vi "html Header.vi"(4 "Test Result":bool, 6 "Test Operator":string="sna001", 7 "Company":string="ELEMASTER", 8 "Serial Numbe (SN)":string="SN123456789", 9 "Hardware Revision":string="v1.1", 10 "Product Info":string="Power Board", 11 "Product Name":string="Safe Torque Off") -> (3 "html string":string="<!DOCTYPE html>\n<html>\n<head>\n<style>\ntable {\n  font-family: arial, sans-serif;\n  border-collapse: collapse;\n  width: 85%;\n}\n\ntd, th {\n  border: 1px solid #dddddd;\n  text-align: left;\n  padding: 8px;\n}\n\ntr:nth-child(even) {\n  background-color: #dddddd;\n}\n</style>\n</head>\n<body>\r<h1 style=\"background-color:Orange; text-align:center; width:85%\">ELEMASTER-Ro: Test Report</h1> \r<h3 style=\"color:Blue\">Under Test (UUT): Info</h3>   \r<table style=\"width: 50%\">  <tr>\n    <th>Company</th>\n    <th>ADB SAFEGATE</th>\n  </tr>  <tr>\n    <td>Product Name</td>\n    <th>ADB LED LMS</th>\n  </tr>  <tr>\n    <td>Product Info</td>\n    <td>LMS Single</td>\n  </tr>  <tr>\n    <td>Hardware Revision</td>\n    <td>v1.1</td>\n  </tr>  <tr>\n    <td>Serial number (SN)</td>\n    <th>sn:12345</th>\n  </tr>  <tr>\n    <td>Test Operator</td>\n    <td>---</td>\n  </tr>  <tr>\n    <td>Date / Time</td>\n    <td>22/09/2021 / 15:30</td>\n  </tr>   <tr>\n    <th>Test Result</th>\n    <th style=\"background-color:Red;color:White\">FALSE</th>\n  </tr></table>\n</body>\n</html>")   [LabVIEW 2018]
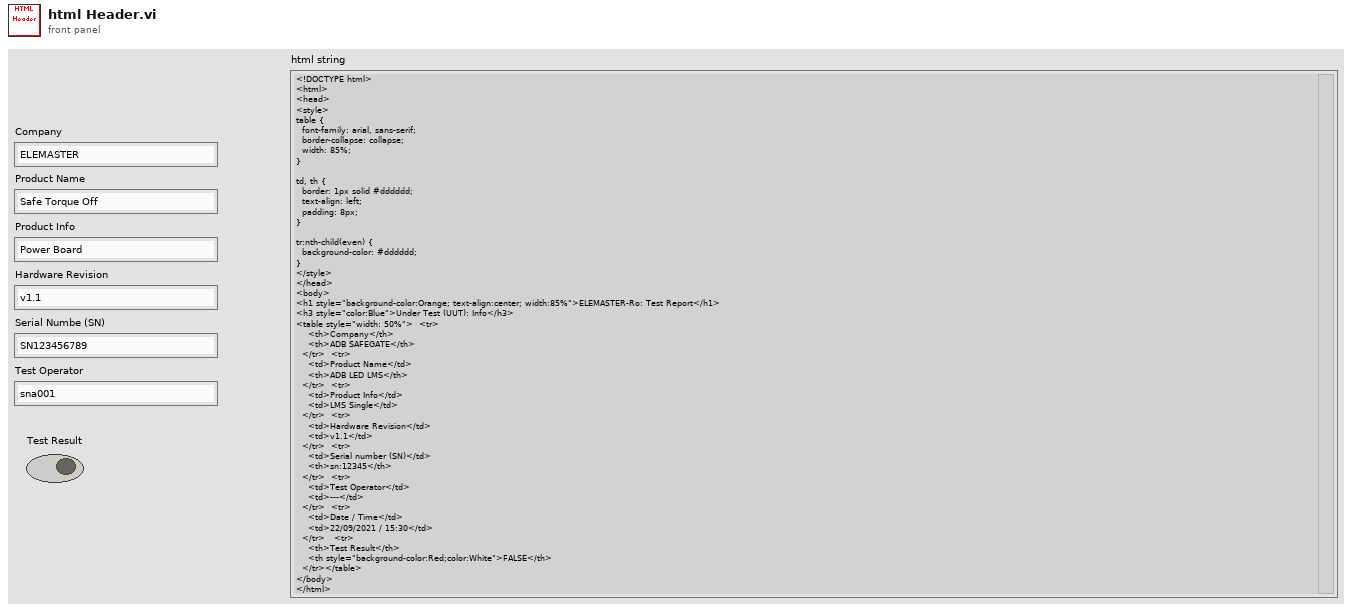
[diagram p1: front panel]
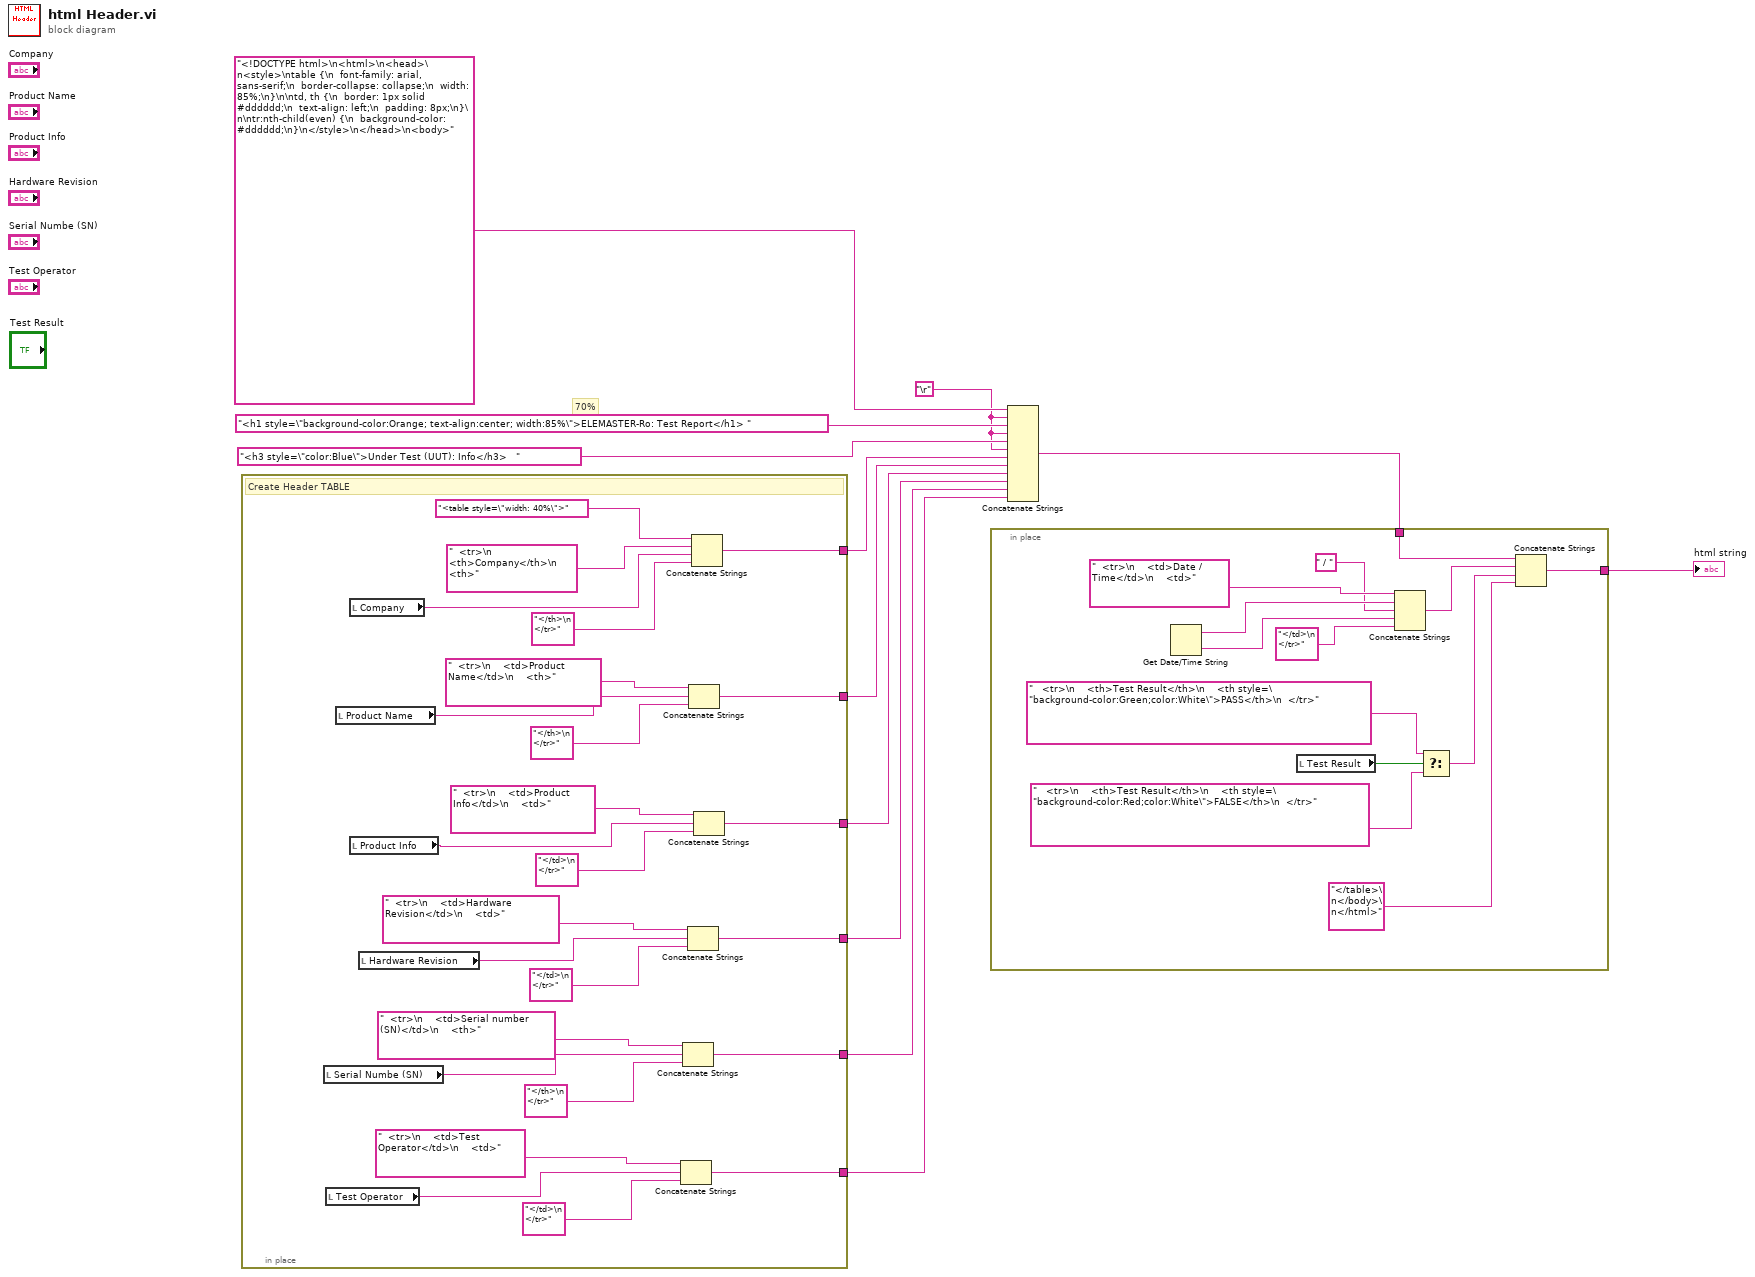
[diagram p0: block diagram]
diagram:
  w7 = "\r"
  # "70%"
  n1 = in-place {
    in-place-border: [w33] -> w6
    in-place-border: [w29] -> w5
    in-place-border: [w16] -> w4
    in-place-border: [w15] -> w3
    in-place-border: [w14] -> w2
    in-place-border: [w13] -> w1
    # "Create Header TABLE"
    n2 = local read "Serial Numbe (SN)"() -> (w20:string)
    n3 = local read "Test Operator"() -> (w17:string)
    n4 = local read "Product Name"() -> (w30:string)
    n5 = local read "Company"() -> (w34:string)
    n6 = local read "Product Info"() -> (w26:string)
    n7 = local read "Hardware Revision"() -> (w23:string)
    n8 = Concatenate Strings("  <tr>\n    <td>Test Operator</td>\n    <td>", w17, "</td>\n  </tr>") -> (w13:string)
    n9 = Concatenate Strings("  <tr>\n    <td>Serial number (SN)</td>\n    <th>", w20, "</th>\n  </tr>") -> (w14:string)
    n10 = Concatenate Strings("  <tr>\n    <td>Hardware Revision</td>\n    <td>", w23, "</td>\n  </tr>") -> (w15:string)
    n11 = Concatenate Strings("  <tr>\n    <td>Product Name</td>\n    <th>", w30, "</th>\n  </tr>") -> (w29:string)
    n12 = Concatenate Strings("<table style=\"width: 40%\">", "  <tr>\n    <th>Company</th>\n    <th>", w34, "</th>\n  </tr>") -> (w33:string)
    n13 = Concatenate Strings("  <tr>\n    <td>Product Info</td>\n    <td>", w26, "</td>\n  </tr>") -> (w16:string)
  }
  n14 = Concatenate Strings("<!DOCTYPE html>\n<html>\n<head>\n<style>\ntable {\n  font-family: arial, sans-serif;\n  border-collapse: collapse;\n  width: 85%;\n}\n\ntd, th {\n  border: 1px solid #dddddd;\n  text-align: left;\n  padding: 8px;\n}\n\ntr:nth-child(even) {\n  background-color: #dddddd;\n}\n</style>\n</head>\n<body>", w7, "<h1 style=\"background-color:Orange; text-align:center; width:85%\">ELEMASTER-Ro: Test Report</h1> ", w7, "<h3 style=\"color:Blue\">Under Test (UUT): Info</h3>   ", w7, w6, w5, w4, w3, w2, w1) -> (w12:string)
  n15 = in-place {
    in-place-border: w12 -> [w50]
    in-place-border: [w49] -> w11
    n16 = Get Date/Time String() -> (date string=w47:string, time string=w45:string)  [unwired: 3 in]
    n17 = local read "Test Result"() -> (w40:bool)
    n18 = Concatenate Strings("  <tr>\n    <td>Date / Time</td>\n    <td>", w47, " / " ("string"), w45, "</td>\n  </tr>") -> (w43:string)
    n19 = Select(t="   <tr>\n    <th>Test Result</th>\n    <th style=\"background-color:Green;color:White\">PASS</th>\n  </tr>", s=w40, f="   <tr>\n    <th>Test Result</th>\n    <th style=\"background-color:Red;color:White\">FALSE</th>\n  </tr>") -> (s? t:f=w39:string)
    n20 = Concatenate Strings(w50, w43, w39, "</table>\n</body>\n</html>") -> (w49:string)
  }
  "html string" <- w11
